vi "CreateCustomDevice.vi"(8 "error in (no error)":errorcluster, 9 "Custom Devices Ref":refnum<k24>, 10 "CD Config Path (.dat)":path, 11 "Name":string) -> (0 "error out":errorcluster, 2 "Custom Devices Ref Out":refnum<k24>, 3 "Node Ptr Out":T1 format="%.0x")   [LabVIEW 2024]
uses:
  NationalInstruments.VeriStand.SystemDefinitionAPI
  <vilib>/NI VeriStand/Custom Device API/Custom Device Item Ref.ctl
  Shared/Constants.vi
  Shared/Embedded TDMS Logger Shared.lvlib
  System Explorer/Embedded TDMS Logger System Explorer.lvlib
  <vilib>/NI VeriStand/Custom Device API/Custom Device API.lvlib
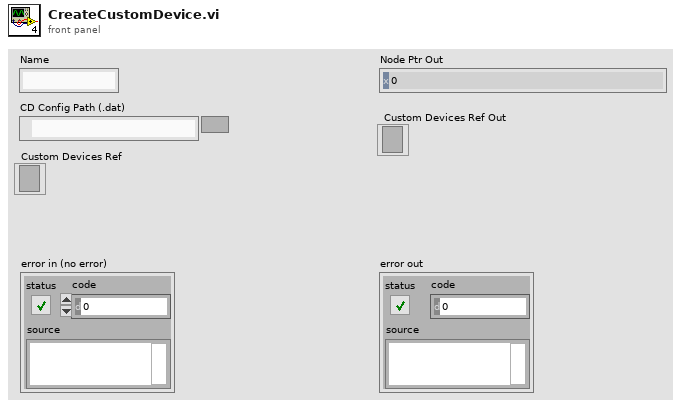
[diagram p1: front panel]
types:
  T1 = typedef "Custom Device API.lvlib/Custom Device Item Ref.ctl" = u64
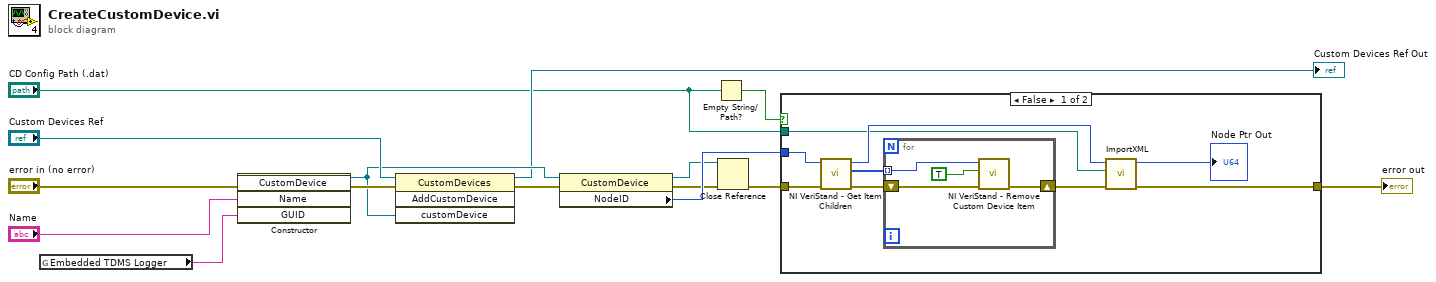
[diagram p0: block diagram]
diagram:
  n1 = global read "Constants.vi" "Embedded TDMS Logger"() -> (w1:string)
  n2 = constructor class="CustomDevice"(error in="error in (no error)", "Name"="Name", "GUID"=w1) -> (reference out=w8:refnum<k24>, error out=w10:errorcluster)  [unwired: 2 in, 3 out]
  n3 = invoke class="CustomDevices" method="AddCustomDevice"(reference="Custom Devices Ref", error in=w10, "customDevice"=w8) -> (reference out=→"Custom Devices Ref Out":refnum<k24>, error out=w9:errorcluster)  [unwired: 1 in, 2 out]
  n4 = property class="CustomDevice"(reference=w8, error in=w9) -> (reference out=w6:refnum<k24>, error out=w5:errorcluster, "NodeID"=w13:u64)
  n5 = Empty String/Path?(string/path="CD Config Path (.dat)") -> (empty?=w2:bool)
  n6 = Close Reference(reference=w6, error in (no error)=w5) -> (error out=w4:errorcluster)
  n7 = case shown="False" w2 {
    tunnel: w13 -> [w19 _]
    tunnel: [w17 w29] -> w12
    tunnel: w4 -> [w20 w29]
    tunnel: "CD Config Path (.dat)" -> [w18 _]
    frame False {
      n8 = call <vilib>:"NI VeriStand - Get Item Children.vi"("error in (no error)"=w20, "Item Ref in"=w19) -> ("error out"=w21:errorcluster, "Child Refs"=w22:T1[], "Item Ref out"=w24:T1)  [unwired: 6 in, 1 out]
      n9 = for {
        shift-right: [w28] -> w23
        shift-left: w21 -> [w27]
        tunnel: w22 -> [w26] mode=indexing
        n10 = call <vilib>:"NI VeriStand - Remove Custom Device Item.vi"("error in (no error)"=w27, "Force Delete (F)"=TRUE, "Item Ref in"=w26) -> ("error out"=w28:errorcluster)  [unwired: 7 in, 1 out]
      }
      n11 = call "ImportXML.vi"("error in (no error)"=w23, "selected path"=w18, "Node Ptr"=w24) -> ("error out"=w17:errorcluster, "Node Ptr Out"=→"Node Ptr Out":T1)  [unwired: 7 in]
    }
    frame True {
    }
  }
  "error out" <- w12
